vi "Prompt Reset.vi"(8 "error in (no error)":errorcluster, 11 "RP2040.lvlib:RP2040Platform in":refnum<class "RP2040Platform.lvclass">) -> (0 "error out":errorcluster, 3 "RP2040.lvlib:RP2040Platform out":refnum<class "RP2040Platform.lvclass">)   [LabVIEW 2020, in "RP2040.lvlib" / "RP2040Platform.lvclass"]
uses:
  RP2040Platform.lvclass
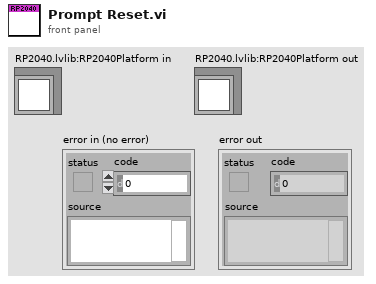
[diagram p1: front panel]
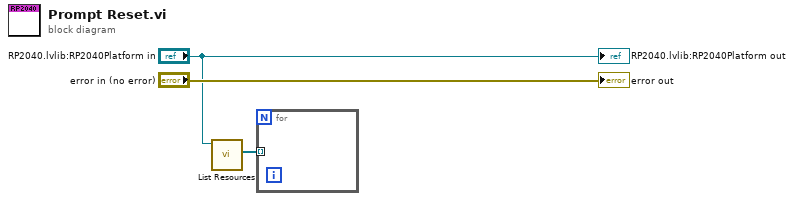
[diagram p0: block diagram]
diagram:
  n1 = call-dynamic "List Resources.vi"("RP2040.lvlib:RP2040Platform in"="RP2040.lvlib:RP2040Platform in") -> ("Resources"=w2:refnum<class "DeployResource.lvclass">[])  [unwired: 8 in, 2 out]
  n2 = for {
    tunnel: w2 -> [_] mode=indexing
  }
  "error out" <- "error in (no error)"
  "RP2040.lvlib:RP2040Platform out" <- "RP2040.lvlib:RP2040Platform in"
